vi "ElevatorStateControl.vi"(9 "Elevator State":string) -> (1 "Elevator State Out":string, 2 "Target Elevator Position":dbl, 4 "Target Vacuum Pump Power":dbl)   [LabVIEW 2018]
uses:
  Inputs_DriverStation.vi
  SensorReadings.vi
  RobotStates.vi
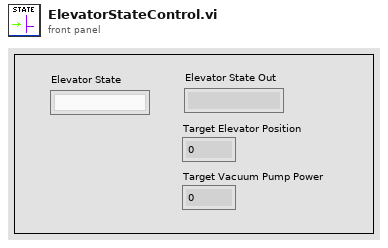
[diagram p1: front panel]
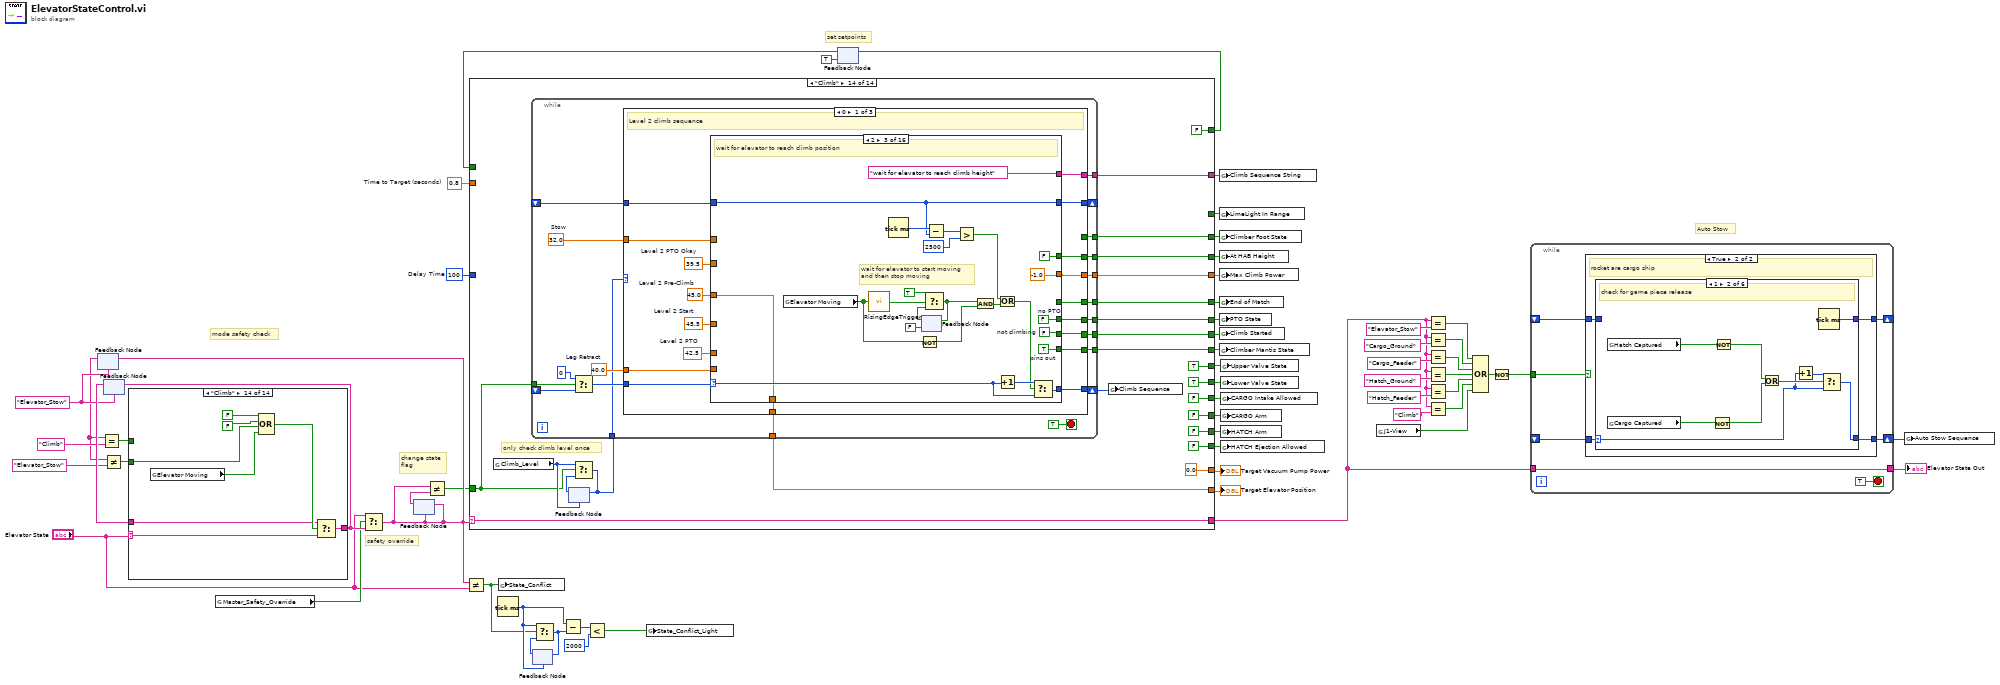
[diagram p0: block diagram]
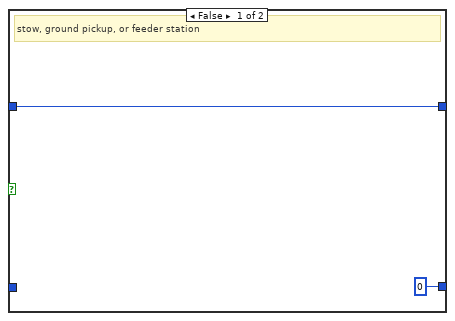
[diagram p2: hidden frame]
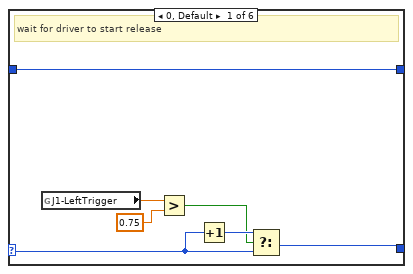
[diagram p3: hidden frame]
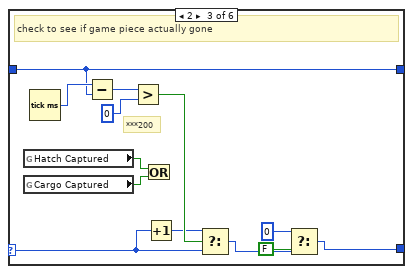
[diagram p4: hidden frame]
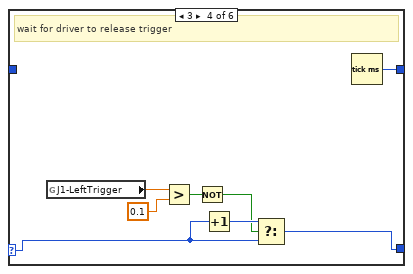
[diagram p5: hidden frame]
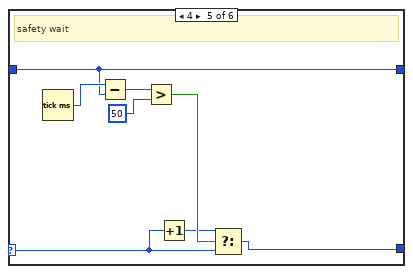
[diagram p6: hidden frame]
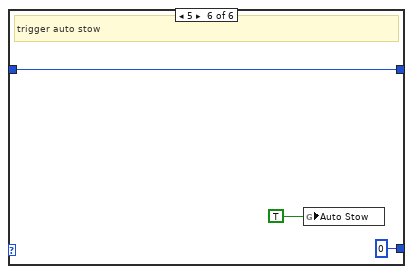
[diagram p7: hidden frame]
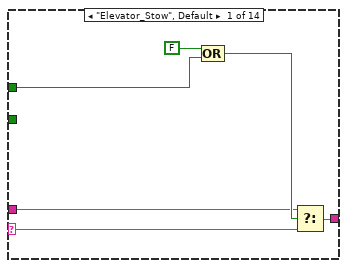
[diagram p8: hidden frame]
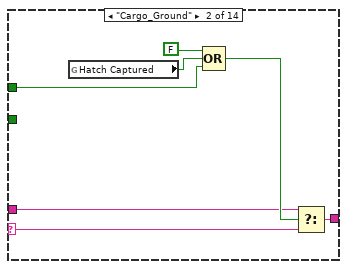
[diagram p9: hidden frame]
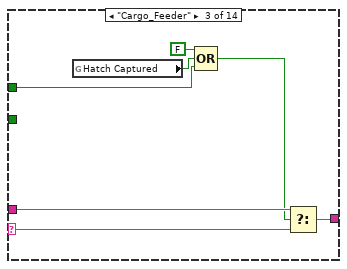
[diagram p10: hidden frame]
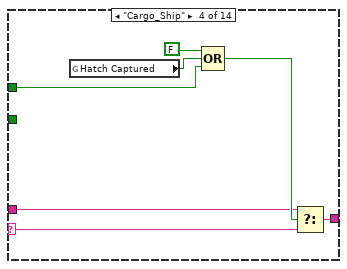
[diagram p11: hidden frame]
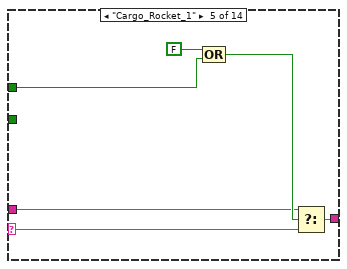
[diagram p12: hidden frame]
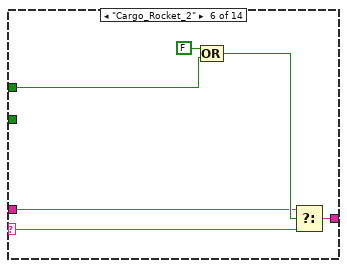
[diagram p13: hidden frame]
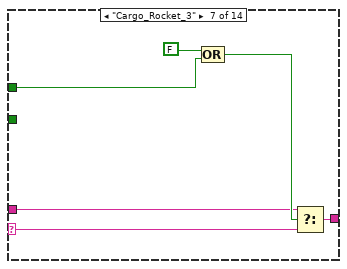
[diagram p14: hidden frame]
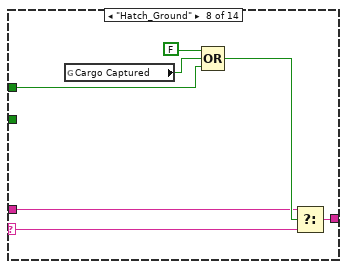
[diagram p15: hidden frame]
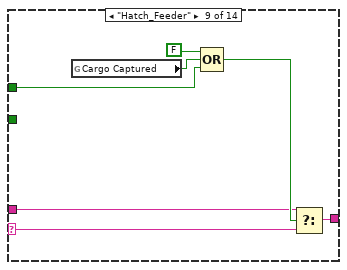
[diagram p16: hidden frame]
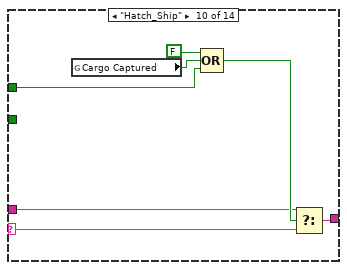
[diagram p17: hidden frame]
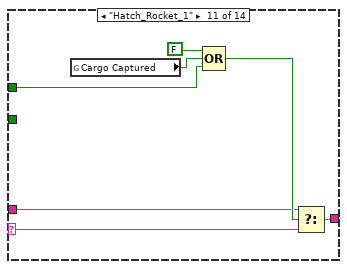
[diagram p18: hidden frame]
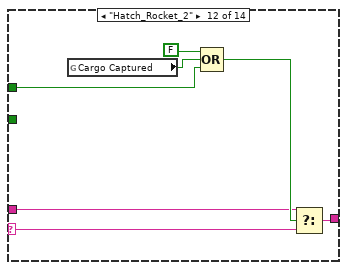
[diagram p19: hidden frame]
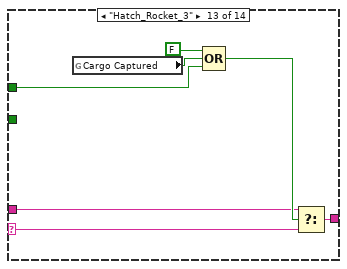
[diagram p20: hidden frame]
diagram:
  w3 = u32 100  # Delay Time
  w4 = 0.8  # Time to Target (seconds)
  w46 = "Elevator_Stow" ("Elevator State")
  # "change state\nflag"
  # "Auto Stow"
  # "safety override"
  # "mode safety check"
  # "set setpoints"
  n1 = feedback #1(w46) -> (w11:string)
  n2 = Equal?(x=w11, y="Climb") -> (x = y?=w47:bool)
  n3 = feedback #2(w46) -> (w49:string)
  n4 = Not Equal?(x=w11, y="Elevator_Stow") -> (x != y?=w10:bool)
  n5 = case shown="\"Climb\"" "Elevator State" {
    selector: "Elevator State" -> [w62 w69 w80 w83 w89 w95 w102 w108 w115 w122 w129 w136 w144 w152]
    tunnel: [w64 w71 w79 w85 w91 w97 w103 w110 w117 w124 w131 w138 w145 w153] -> w54
    tunnel: w49 -> [w63 w70 w78 w84 w90 w96 w101 w109 w116 w123 w130 w137 w143 w151]
    tunnel: w47 -> [w61 w67 w74 w81 w88 w94 w100 w106 w113 w120 w127 w134 w141 _]
    tunnel: w10 -> [_ _ _ _ _ _ _ _ _ _ _ _ _ w150]
    frame "Elevator_Stow", Default {
      n6 = Compound Arithmetic op=OR(FALSE, w61) -> (w65:bool)
      n7 = Select(t=w63, s=w65, f=w62) -> (s? t:f=w64:string)
    }
    frame "Cargo_Ground" {
      n8 = global read "SensorReadings.vi" "Hatch Captured"() -> (w68:bool)
      n9 = Compound Arithmetic op=OR(FALSE, w68, w67) -> (w72:bool)
      n10 = Select(t=w70, s=w72, f=w69) -> (s? t:f=w71:string)
    }
    frame "Cargo_Feeder" {
      n11 = global read "SensorReadings.vi" "Hatch Captured"() -> (w75:bool)
      n12 = Compound Arithmetic op=OR(FALSE, w75, w74) -> (w76:bool)
      n13 = Select(t=w78, s=w76, f=w80) -> (s? t:f=w79:string)
    }
    frame "Cargo_Ship" {
      n14 = global read "SensorReadings.vi" "Hatch Captured"() -> (w82:bool)
      n15 = Compound Arithmetic op=OR(FALSE, w82, w81) -> (w86:bool)
      n16 = Select(t=w84, s=w86, f=w83) -> (s? t:f=w85:string)
    }
    frame "Cargo_Rocket_1" {
      n17 = Compound Arithmetic op=OR(FALSE, w88) -> (w92:bool)
      n18 = Select(t=w90, s=w92, f=w89) -> (s? t:f=w91:string)
    }
    frame "Cargo_Rocket_2" {
      n19 = Compound Arithmetic op=OR(FALSE, w94) -> (w98:bool)
      n20 = Select(t=w96, s=w98, f=w95) -> (s? t:f=w97:string)
    }
    frame "Cargo_Rocket_3" {
      n21 = Compound Arithmetic op=OR(FALSE, w100) -> (w104:bool)
      n22 = Select(t=w101, s=w104, f=w102) -> (s? t:f=w103:string)
    }
    frame "Hatch_Ground" {
      n23 = global read "SensorReadings.vi" "Cargo Captured"() -> (w107:bool)
      n24 = Compound Arithmetic op=OR(FALSE, w107, w106) -> (w111:bool)
      n25 = Select(t=w109, s=w111, f=w108) -> (s? t:f=w110:string)
    }
    frame "Hatch_Feeder" {
      n26 = global read "SensorReadings.vi" "Cargo Captured"() -> (w114:bool)
      n27 = Compound Arithmetic op=OR(FALSE, w114, w113) -> (w118:bool)
      n28 = Select(t=w116, s=w118, f=w115) -> (s? t:f=w117:string)
    }
    frame "Hatch_Ship" {
      n29 = global read "SensorReadings.vi" "Cargo Captured"() -> (w121:bool)
      n30 = Compound Arithmetic op=OR(FALSE, w121, w120) -> (w125:bool)
      n31 = Select(t=w123, s=w125, f=w122) -> (s? t:f=w124:string)
    }
    frame "Hatch_Rocket_1" {
      n32 = global read "SensorReadings.vi" "Cargo Captured"() -> (w128:bool)
      n33 = Compound Arithmetic op=OR(FALSE, w128, w127) -> (w132:bool)
      n34 = Select(t=w130, s=w132, f=w129) -> (s? t:f=w131:string)
    }
    frame "Hatch_Rocket_2" {
      n35 = global read "SensorReadings.vi" "Cargo Captured"() -> (w135:bool)
      n36 = Compound Arithmetic op=OR(FALSE, w135, w134) -> (w139:bool)
      n37 = Select(t=w137, s=w139, f=w136) -> (s? t:f=w138:string)
    }
    frame "Hatch_Rocket_3" {
      n38 = global read "SensorReadings.vi" "Cargo Captured"() -> (w142:bool)
      n39 = Compound Arithmetic op=OR(FALSE, w142, w141) -> (w146:bool)
      n40 = Select(t=w143, s=w146, f=w144) -> (s? t:f=w145:string)
    }
    frame "Climb" {
      n41 = global read "RobotStates.vi" "Elevator Moving"() -> (w149:bool)
      n42 = Compound Arithmetic op=OR(FALSE, FALSE ("Cargo Captured"), w150, w149) -> (w154:bool)
      n43 = Select(t=w151, s=w154, f=w152) -> (s? t:f=w153:string)
    }
  }
  n44 = feedback-in #2(w54) -> ()
  n45 = global read "Inputs_DriverStation.vi" "Master_Safety_Override"() -> (w53:bool)
  n46 = Select(t="Elevator State", s=w53, f=w54) -> (s? t:f=w16:string)
  n47 = feedback-in #1(w16) -> ()
  n48 = feedback-in #3(w16) -> ()
  n49 = feedback #3(w16) -> (w17:string)
  n50 = Not Equal?(x=w16, y=w17) -> (x != y?=w15:bool)
  n51 = Not Equal?(x=w16, y="Elevator State") -> (x != y?=w22:bool)
  n52 = Tick Count (ms)() -> (millisecond timer value=w26:u32)
  n53 = global write "RobotStates.vi" "State_Conflict"(w22) -> ()
  n54 = feedback #4(w26) -> (w27:u32)
  n55 = Select(t=w26, s=w22, f=w27) -> (s? t:f=w25:u32)
  n56 = feedback-in #4(w25) -> ()
  n57 = Subtract(x=w26, y=w25) -> (x-y=w24:u32)
  n58 = Less?(x=w24, y=u32 2000) -> (x < y?=w21:bool)
  n59 = global write "RobotStates.vi" "State_Conflict_Light"(w21) -> ()
  n60 = feedback #5(TRUE) -> (w19:bool)
  n61 = case shown="\"Climb\"" w16 {
    selector: w16 -> [w179 w194 w234 w252 w293 w315 w337 w351 w413 w454 w495 w510 w525 w550]
    tunnel: [FALSE TRUE TRUE TRUE TRUE TRUE TRUE FALSE FALSE FALSE FALSE FALSE FALSE FALSE] -> w60
    tunnel: [w179 w194 w234 w252 w293 w315 w337 w351 w413 w454 w495 w510 w525 w550] -> w29
    tunnel: [w157 FALSE w197 w235 TRUE w296 w319 FALSE FALSE FALSE FALSE FALSE FALSE FALSE] -> w59
    tunnel: [w178 32.0 w204 w236 w279 w300 w317 32.0 w378 w440 w481 61.5 91.0 w536] -> w58
    tunnel: [FALSE FALSE FALSE FALSE FALSE FALSE FALSE TRUE w382 TRUE TRUE TRUE TRUE FALSE] -> w57
    tunnel: [w170 0.0 0.0 0.0 0.0 0.0 0.0 w347 w411 w452 w493 w506 w521 0.0 ("Vacuum_Pump")] -> w55
    tunnel: [FALSE FALSE FALSE FALSE FALSE FALSE FALSE TRUE TRUE TRUE TRUE TRUE TRUE FALSE] -> w56
    tunnel: [TRUE TRUE TRUE TRUE TRUE TRUE TRUE TRUE FALSE FALSE FALSE FALSE FALSE TRUE] -> w52
    tunnel: [TRUE TRUE TRUE TRUE TRUE TRUE TRUE FALSE TRUE TRUE TRUE TRUE TRUE TRUE] -> w51
    tunnel: [FALSE FALSE FALSE FALSE FALSE FALSE FALSE FALSE FALSE FALSE FALSE FALSE FALSE w539] -> w1
    tunnel: [w168 FALSE FALSE FALSE FALSE FALSE FALSE FALSE FALSE FALSE FALSE FALSE FALSE FALSE] -> w20
    tunnel: w19 -> [w164 _ _ _ _ _ _ _ _ _ _ _ _ _]
    tunnel: w15 -> [_ _ w212 _ _ _ _ _ w384 _ _ _ _ w538]
    tunnel: [w167 w184 w203 w244 w284 w307 w329 w342 w390 w447 w488 w501 w516 w535] -> w14
    tunnel: [w166 w183 w202 w243 w283 w306 w328 w341 w389 w446 w487 w500 w515 w534] -> w13
    tunnel: [FALSE FALSE FALSE FALSE FALSE FALSE FALSE FALSE FALSE FALSE FALSE FALSE FALSE w533] -> w9
    tunnel: [_ _ _ _ _ _ _ _ _ _ _ _ _ w531] -> w8
    tunnel: [-1.0 ("y") -1.0 ("y") -1.0 ("y") -1.0 ("y") -1.0 ("y") -1.0 ("y") -1.0 ("y") -1.0 ("y") -1.0 ("y") -1.0 ("y") -1.0 ("y") -1.0 ("y") -1.0 ("y") w530] -> w7
    tunnel: [_ _ _ _ _ _ _ _ _ _ _ _ _ w529] -> w6
    tunnel: [_ _ _ _ w271 _ _ _ w371 w433 w474 _ _ _] -> w5
    tunnel: w4 -> [_ _ _ _ w269 _ _ _ w369 w432 w472 _ _ _]
    tunnel: w3 -> [_ _ _ _ w270 _ _ _ w370 w431 w473 _ _ _]
    tunnel: [_ _ _ _ _ _ _ _ _ _ _ _ _ w528] -> w2
    frame "Elevator_Stow", Default {
      w166 = FALSE  # no PTO
      w167 = FALSE  # not climbing
      w178 = 30.0  # below 34.5 to ensure reset
      n62 = global read "Inputs_DriverStation.vi" "Reinit_Stow_Vacuum"() -> (w161:bool)
      n63 = global read "Inputs_DriverStation.vi" "Vacuum_Pump"() -> (w172:dbl)
      n64 = global read "RobotStates.vi" "Autopilot"() -> (w160:bool)
      n65 = Select(t=TRUE, s=w161, f=w164) -> (s? t:f=w163:bool)
      n66 = Select(t=w172, s=w163, f=0.0) -> (s? t:f=w170:dbl)
      n67 = Select(t=TRUE, s=w163, f=w163) -> (s? t:f=w168:bool)
      n68 = Select(t=TRUE, s=w160, f=FALSE) -> (s? t:f=w157:bool)
    }
    frame "Cargo_Ground" {
      w183 = FALSE  # no PTO
      w184 = FALSE  # not climbing
    }
    frame "Cargo_Feeder" {
      w199 = TRUE  # hold CARGO arm up
      w202 = FALSE  # no PTO
      w203 = FALSE  # not climbing
      w205 = 32.0  # gotten CARGO
      w209 = FALSE  # gotten CARGO
      w221 = -2.0  # (ft/s)
      w208 = 52.0  # getting CARGO
      w210 = TRUE  # getting CARGO
      # "autopilot"
      # "auto protect CARGO"
      n69 = global read "SensorReadings.vi" "EncoderVel_RightDrive"() -> (w225:dbl)
      n70 = global read "SensorReadings.vi" "EncoderVel_LeftDrive"() -> (w226:dbl)
      n71 = global read "SensorReadings.vi" "Cargo Captured"() -> (w219:bool)
      n72 = Add(x=w226, y=w225) -> (x+y=w224:dbl)
      n73 = Divide(x=w224, y=2.0) -> (x/y=w222:dbl)
      n74 = Less?(x=w222, y=w221) -> (x < y?=w220:bool)
      n75 = And(x=w220, y=w219) -> (x .and. y?=w218:bool)
      n76 = feedback #6(FALSE) -> (w216:bool)
      n77 = Select(t=TRUE, s=w218, f=w216) -> (s? t:f=w214:bool)
      n78 = Select(t=FALSE, s=w212, f=w214) -> (s? t:f=w207:bool)
      n79 = feedback-in #6(w207) -> ()
      n80 = Not(x=w207) -> (.not. x?=w206:bool)
      n81 = global read "RobotStates.vi" "Autopilot"() -> (w200:bool)
      n82 = Select(t=w210, s=w206, f=w209) -> (s? t:f=w198:bool)
      n83 = Select(t=w199, s=w200, f=w198) -> (s? t:f=w197:bool)
      n84 = Select(t=w208, s=w206, f=w205) -> (s? t:f=w204:dbl)
    }
    frame "Cargo_Ship" {
      w243 = FALSE  # no PTO
      w244 = FALSE  # not climbing
      w236 = 48.0
      # "46"
      n85 = global read "SensorReadings.vi" "EncoderPos_Elevator"() -> (w240:dbl)
      n86 = Subtract(x=w240, y=w236) -> (x-y=w239:dbl)
      n87 = Absolute Value(x=w239) -> (abs(x)=w237:dbl)
      n88 = Less?(x=w237, y=5.0) -> (x < y?=w235:bool)
    }
    frame "Cargo_Rocket_1" {
      w260 = 3.0  # feet per second
      w283 = FALSE  # no PTO
      w284 = FALSE  # not climbing
      n89 = global read "SensorReadings.vi" "LimeLight Distance (in)"() -> (w258:dbl)
      n90 = global read "SensorReadings.vi" "EncoderVel_RightDrive"() -> (w267:dbl)
      n91 = global read "SensorReadings.vi" "EncoderVel_LeftDrive"() -> (w268:dbl)
      n92 = Add(x=w268, y=w267) -> (x+y=w266:dbl)
      n93 = Divide(x=w258, y=12.0) -> (x/y=w256:dbl)
      n94 = Divide(x=w266, y=2.0) -> (x/y=w261:dbl)
      n95 = In Range and Coerce(upper limit=10.0, x=w261, lower limit=w260) -> (coerced(x)=w259:dbl)  [unwired: 1 out]
      n96 = Divide(x=w256, y=w259) -> (x/y=w263:dbl)
      n97 = Greater Than 0?(x=w263) -> (x > 0?=w264:bool)
      n98 = Select(t=w263, s=w264, f=inf) -> (s? t:f=w255:dbl)
      n99 = global read "SensorReadings.vi" "LimeLight Valid"() -> (w274:bool)
      n100 = Select(t=w255, s=w274, f=inf) -> (s? t:f=w273:dbl)
      n101 = call "TimeBelowThreshold.vi"("Current Value"=w273, "Threshold"=w269) -> ("Time Below"=w275:u32)  [unwired: 3 in]
      n102 = global read "RobotStates.vi" "Autopilot"() -> (w281:bool)
      n103 = Greater?(x=w275, y=w270) -> (0:w276:bool)
      n104 = call "RisingEdgeTrigger.vi"("Raw Signal"=w276) -> ("Trigger"=w271:bool)
      n105 = Select(t=45.0, s=w281, f=32.0) -> (s? t:f=w279:dbl)
    }
    frame "Cargo_Rocket_2" {
      w306 = FALSE  # no PTO
      w307 = FALSE  # not climbing
      w300 = 62.5
      n106 = global read "SensorReadings.vi" "EncoderPos_Elevator"() -> (w301:dbl)
      n107 = Subtract(x=w301, y=w300) -> (x-y=w299:dbl)
      n108 = Absolute Value(x=w299) -> (abs(x)=w295:dbl)
      n109 = Less?(x=w295, y=10.0) -> (x < y?=w297:bool)
      n110 = Select(t=TRUE, s=w297, f=FALSE) -> (s? t:f=w296:bool)
    }
    frame "Cargo_Rocket_3" {
      w328 = FALSE  # no PTO
      w329 = FALSE  # not climbing
      w317 = 91.0
      n111 = global read "SensorReadings.vi" "EncoderPos_Elevator"() -> (w323:dbl)
      n112 = Subtract(x=w323, y=w317) -> (x-y=w322:dbl)
      n113 = Absolute Value(x=w322) -> (abs(x)=w320:dbl)
      n114 = Less?(x=w320, y=10.0) -> (x < y?=w321:bool)
      n115 = Select(t=TRUE, s=w321, f=FALSE) -> (s? t:f=w319:bool)
    }
    frame "Hatch_Ground" {
      w341 = FALSE  # no PTO
      w342 = FALSE  # not climbing
      n116 = global read "Inputs_DriverStation.vi" "Vacuum_Pump"() -> (w347:dbl)
    }
    frame "Hatch_Feeder" {
      w359 = 3.0  # feet per second
      w389 = FALSE  # no PTO
      w390 = FALSE  # not climbing
      w400 = -2.0  # (ft/s)
      w392 = FALSE  # gotten HATCH
      w406 = TRUE  # to get HATCH
      # "auto protect HATCH"
      n117 = global read "SensorReadings.vi" "EncoderVel_RightDrive"() -> (w404:dbl)
      n118 = global read "SensorReadings.vi" "EncoderVel_LeftDrive"() -> (w405:dbl)
      n119 = global read "SensorReadings.vi" "LimeLight Distance (in)"() -> (w357:dbl)
      n120 = global read "SensorReadings.vi" "EncoderVel_RightDrive"() -> (w367:dbl)
      n121 = global read "SensorReadings.vi" "EncoderVel_LeftDrive"() -> (w368:dbl)
      n122 = global read "SensorReadings.vi" "Hatch Captured"() -> (w386:bool)
      n123 = Add(x=w405, y=w404) -> (x+y=w403:dbl)
      n124 = Divide(x=w403, y=2.0) -> (x/y=w401:dbl)
      n125 = Less?(x=w401, y=w400) -> (x < y?=w399:bool)
      n126 = Add(x=w368, y=w367) -> (x+y=w366:dbl)
      n127 = And(x=w399, y=w386) -> (x .and. y?=w398:bool)
      n128 = Not(x=w386) -> (.not. x?=w385:bool)
      n129 = Divide(x=w357, y=12.0) -> (x/y=w355:dbl)
      n130 = Divide(x=w366, y=2.0) -> (x/y=w360:dbl)
      n131 = Or(x=w385, y=w384) -> (x .or. y?=w383:bool)
      n132 = feedback #7(FALSE) -> (w396:bool)
      n133 = Select(t=TRUE, s=w398, f=w396) -> (s? t:f=w394:bool)
      n134 = In Range and Coerce(upper limit=10.0 ("feet per second"), x=w360, lower limit=w359) -> (coerced(x)=w358:dbl)  [unwired: 1 out]
      n135 = Select(t=FALSE, s=w383, f=w394) -> (s? t:f=w391:bool)
      n136 = feedback-in #7(w391) -> ()
      n137 = Divide(x=w355, y=w358) -> (x/y=w363:dbl)
      n138 = Not(x=w391) -> (.not. x?=w387:bool)
      n139 = Greater Than 0?(x=w363) -> (x > 0?=w364:bool)
      n140 = Select(t=w363, s=w364, f=inf) -> (s? t:f=w361:dbl)
      n141 = global read "SensorReadings.vi" "LimeLight Valid"() -> (w375:bool)
      n142 = Select(t=w406, s=w387, f=w392) -> (s? t:f=w382:bool)
      n143 = Select(t=w361, s=w375, f=inf) -> (s? t:f=w376:dbl)
      n144 = global read "RobotStates.vi" "Autopilot"() -> (w381:bool)
      n145 = call "TimeBelowThreshold.vi"("Current Value"=w376, "Threshold"=w369) -> ("Time Below"=w373:u32)  [unwired: 3 in]
      n146 = global read "Inputs_DriverStation.vi" "Vacuum_Pump"() -> (w411:dbl)
      n147 = Greater?(x=w373, y=w370) -> (0:w372:bool)
      n148 = Select(t=55.0, s=w381, f=32.0) -> (s? t:f=w378:dbl)
      n149 = call "RisingEdgeTrigger.vi"("Raw Signal"=w372) -> ("Trigger"=w371:bool)
    }
    frame "Hatch_Ship" {
      w422 = 3.0  # feet per second
      w446 = FALSE  # no PTO
      w447 = FALSE  # not climbing
      n150 = global read "SensorReadings.vi" "LimeLight Distance (in)"() -> (w420:dbl)
      n151 = global read "SensorReadings.vi" "EncoderVel_RightDrive"() -> (w429:dbl)
      n152 = global read "SensorReadings.vi" "EncoderVel_LeftDrive"() -> (w430:dbl)
      n153 = Add(x=w430, y=w429) -> (x+y=w428:dbl)
      n154 = Divide(x=w420, y=12.0) -> (x/y=w418:dbl)
      n155 = Divide(x=w428, y=2.0) -> (x/y=w423:dbl)
      n156 = In Range and Coerce(upper limit=10.0, x=w423, lower limit=w422) -> (coerced(x)=w421:dbl)  [unwired: 1 out]
      n157 = Divide(x=w418, y=w421) -> (x/y=w425:dbl)
      n158 = Greater Than 0?(x=w425) -> (x > 0?=w426:bool)
      n159 = Select(t=w425, s=w426, f=inf) -> (s? t:f=w417:dbl)
      n160 = global read "SensorReadings.vi" "LimeLight Valid"() -> (w437:bool)
      n161 = Select(t=w417, s=w437, f=inf) -> (s? t:f=w438:dbl)
      n162 = call "TimeBelowThreshold.vi"("Current Value"=w438, "Threshold"=w432) -> ("Time Below"=w435:u32)  [unwired: 3 in]
      n163 = global read "RobotStates.vi" "Autopilot"() -> (w443:bool)
      n164 = global read "Inputs_DriverStation.vi" "Vacuum_Pump"() -> (w452:dbl)
      n165 = Greater?(x=w435, y=w431) -> (0:w434:bool)
      n166 = call "RisingEdgeTrigger.vi"("Raw Signal"=w434) -> ("Trigger"=w433:bool)
      n167 = Select(t=55.0, s=w443, f=32.0) -> (s? t:f=w440:dbl)
    }
    frame "Hatch_Rocket_1" {
      w463 = 3.0  # feet per second
      w487 = FALSE  # no PTO
      w488 = FALSE  # not climbing
      # "autopilot"
      n168 = global read "SensorReadings.vi" "LimeLight Distance (in)"() -> (w461:dbl)
      n169 = global read "SensorReadings.vi" "EncoderVel_RightDrive"() -> (w470:dbl)
      n170 = global read "SensorReadings.vi" "EncoderVel_LeftDrive"() -> (w471:dbl)
      n171 = Add(x=w471, y=w470) -> (x+y=w469:dbl)
      n172 = Divide(x=w461, y=12.0) -> (x/y=w459:dbl)
      n173 = Divide(x=w469, y=2.0) -> (x/y=w464:dbl)
      n174 = In Range and Coerce(upper limit=10.0, x=w464, lower limit=w463) -> (coerced(x)=w462:dbl)  [unwired: 1 out]
      n175 = Divide(x=w459, y=w462) -> (x/y=w466:dbl)
      n176 = Greater Than 0?(x=w466) -> (x > 0?=w467:bool)
      n177 = Select(t=w466, s=w467, f=inf) -> (s? t:f=w458:dbl)
      n178 = global read "SensorReadings.vi" "LimeLight Valid"() -> (w477:bool)
      n179 = Select(t=w458, s=w477, f=inf) -> (s? t:f=w476:dbl)
      n180 = call "TimeBelowThreshold.vi"("Current Value"=w476, "Threshold"=w472) -> ("Time Below"=w478:u32)  [unwired: 3 in]
      n181 = Greater?(x=w478, y=w473) -> (0:w479:bool)
      n182 = global read "RobotStates.vi" "Autopilot"() -> (w484:bool)
      n183 = global read "Inputs_DriverStation.vi" "Vacuum_Pump"() -> (w493:dbl)
      n184 = call "RisingEdgeTrigger.vi"("Raw Signal"=w479) -> ("Trigger"=w474:bool)
      n185 = Select(t=55.0, s=w484, f=32.0) -> (s? t:f=w481:dbl)
    }
    frame "Hatch_Rocket_2" {
      w500 = FALSE  # no PTO
      w501 = FALSE  # not climbing
      n186 = global read "Inputs_DriverStation.vi" "Vacuum_Pump"() -> (w506:dbl)
    }
    frame "Hatch_Rocket_3" {
      w515 = FALSE  # no PTO
      w516 = FALSE  # not climbing
      n187 = global read "Inputs_DriverStation.vi" "Vacuum_Pump"() -> (w521:dbl)
    }
    frame "Climb" {
      # "only check climb level once"
      n188 = global read "Inputs_DriverStation.vi" "Climb_Level"() -> (w540:u8)
      n189 = feedback #8(w540) -> (w541:u8)
      n190 = Select(t=w540, s=w538, f=w541) -> (s? t:f=w537:u8)
      n191 = while {
        shift-right: [w569] -> w532
        shift-left: _ -> [w565]
        shift-right: [w568] -> _
        shift-left: _ -> [w567]
        tunnel: [w566] -> w539
        tunnel: w538 -> [w563]
        tunnel: w537 -> [w556]
        tunnel: [w558] -> w536
        tunnel: [w561] -> w535
        tunnel: [w560] -> w534
        tunnel: [w559] -> w533
        tunnel: [w555] -> w531
        tunnel: [w554] -> w530
        tunnel: [w553] -> w529
        tunnel: [w551] -> w528
        stop <- TRUE stop-if-true
        w552 = 32.0  # Stow
        w557 = 40.0  # Leg Retract
        n192 = Select(t=0, s=w563, f=w565) -> (s? t:f=w564:i32)
        n193 = case shown="0" w556 {
          tunnel: [w582 w841 w1064] -> w569
          tunnel: [w586 w848 w1071] -> w568
          tunnel: w567 -> [w588 w849 w1072]
          tunnel: [w581 w842 w1065] -> w566
          tunnel: w564 -> [w584 w847 w1070]
          tunnel: [w579 w843 w1066] -> w561
          tunnel: [w580 w844 w1067] -> w560
          tunnel: [w583 w845 w1068] -> w559
          tunnel: [w578 w840 w1063] -> w558
          tunnel: w557 -> [w585 w846 w1069]
          tunnel: [w587 w839 w1062] -> w555
          tunnel: [w577 w837 w1060] -> w554
          tunnel: [w576 w835 w1058] -> w553
          tunnel: w552 -> [w571 w834 w1057]
          tunnel: [_ _ w1056] -> w551
          frame 0 {
            w575 = 45.0  # Level 2 Pre-Climb
            w572 = 39.5  # Level 2 PTO Okay
            w574 = 45.5  # Level 2 Start
            w573 = 42.5  # Level 2 PTO
            # "Level 2 climb sequence"
            n194 = case shown="2" w584 {
              selector: w584 -> [w598 w614 w634 w651 w662 w683 w694 w713 w732 w743 w761 w770 w785 w797 w814 w828]
              tunnel: [w600 w616 w630 w650 w661 w682 w696 w715 w731 w742 w760 w769 w784 w796 w813 w828] -> w582
              tunnel: [w597 w601 w620 w648 w664 w675 w695 w714 w727 w735 w748 w773 w787 w799 w821 w831] -> w586
              tunnel: w588 -> [_ w604 w620 _ w664 w675 w695 w714 w727 _ w748 w773 w787 w799 w821 w831]
              tunnel: [w596 w613 w640 w649 w660 w685 w699 w718 w734 w745 w763 w774 w788 w800 w822 w832] -> w581
              tunnel: [w589 w602 w624 w641 w653 w668 _ w703 _ _ _ _ w780 w795 w816 w825] -> w578
              tunnel: [w594 w612 w629 w646 w659 w678 w700 w719 w730 w741 w759 w775 w789 w801 w823 w833] -> w579
              tunnel: [w593 w611 w628 w645 w658 w677 w701 w720 w729 w740 w758 w768 w783 w793 w819 w829] -> w580
              tunnel: [FALSE FALSE FALSE FALSE FALSE FALSE FALSE FALSE FALSE FALSE FALSE w772 TRUE TRUE TRUE FALSE] -> w583
              tunnel: w585 -> [_ _ _ _ _ _ _ _ _ _ _ _ w780 w795 w816 w825]
              tunnel: ["release mantis" "wait for mantis to deploy" "wait for elevator to reach climb height" "lock mantis" "confirm mantis lock" "wait for the driver to start climbing #1" "wait for driver to raise elevator" "wait for elevator to reach start height" "wait for elevator to pass PTO height" "engage the PTO" "ensure PTO is engaged" "wait for the robot to be on HAB" "stop climbing" "wait to disengage PTO" "retract the legs after confirm " "elevator powered down"] -> w587
              tunnel: [-1.0 ("y") -1.0 ("y") -1.0 ("y") -1.0 ("y") -1.0 ("y") -1.0 ("y") -1.0 ("y") -1.0 ("y") -0.05 ("y") -0.05 ("y") -0.05 ("y") -1.0 ("y") -1.0 ("y") -1.0 ("y") -1.0 ("y") -1.0 ("y")] -> w577
              tunnel: [_ _ _ _ _ _ _ _ _ _ _ _ _ _ _ w824] -> w576
              tunnel: w575 -> [_ _ w624 w641 w653 w668 _ _ _ _ _ _ _ _ _ _]
              tunnel: w574 -> [_ _ _ _ _ _ _ w703 _ _ _ _ _ _ _ _]
              tunnel: w573 -> [_ _ _ _ _ _ _ _ w722 _ _ _ _ _ _ _]
              tunnel: w572 -> [_ _ _ _ _ _ _ _ _ _ w746 _ _ _ _ _]
              tunnel: w571 -> [w589 w602 _ _ _ _ _ _ _ _ _ _ _ _ _ _]
              frame 0, Default {
                w593 = FALSE  # no PTO
                w594 = FALSE  # not climbing
                w596 = TRUE  # pins out
                # "release mantis pins and command to climb height"
                n195 = Increment(x=w598) -> (x+1=w599:i32)
                n196 = Select(t=w599, s=TRUE, f=w598) -> (s? t:f=w600:i32)
                n197 = Tick Count (ms)() -> (millisecond timer value=w597:u32)
              }
              frame 1 {
                w611 = FALSE  # no PTO
                w612 = FALSE  # not climbing
                w613 = TRUE  # pins out
                # "wait for mantis to deploy"
                n198 = Tick Count (ms)() -> (millisecond timer value=w607:u32)
                n199 = Subtract(x=w607, y=w604) -> (x-y=w606:u32)
                n200 = Greater?(x=w606, y=u32 0) -> (0:w603:bool)
                n201 = Increment(x=w614) -> (x+1=w615:i32)
                n202 = Select(t=w615, s=w603, f=w614) -> (s? t:f=w616:i32)
                n203 = Tick Count (ms)() -> (millisecond timer value=w601:u32)
              }
              frame 2 {
                w628 = FALSE  # no PTO
                w629 = FALSE  # not climbing
                w640 = TRUE  # pins out
                # "wait for elevator to start moving\nand then stop moving"
                # "wait for elevator to reach climb position"
                n204 = global read "RobotStates.vi" "Elevator Moving"() -> (w632:bool)
                n205 = call "RisingEdgeTrigger.vi"("Raw Signal"=w632) -> ("Trigger"=w639:bool)
                n206 = Tick Count (ms)() -> (millisecond timer value=w623:u32)
                n207 = Not(x=w632) -> (.not. x?=w631:bool)
                n208 = feedback #9(FALSE) -> (w637:bool)
                n209 = Select(t=TRUE, s=w639, f=w637) -> (s? t:f=w633:bool)
                n210 = feedback-in #9(w633) -> ()
                n211 = Subtract(x=w623, y=w620) -> (x-y=w622:u32)
                n212 = Greater?(x=w622, y=u32 2500) -> (0:w617:bool)
                n213 = And(x=w633, y=w631) -> (x .and. y?=w619:bool)
                n214 = Or(x=w617, y=w619) -> (x .or. y?=w618:bool)
                n215 = Increment(x=w634) -> (x+1=w635:i32)
                n216 = Select(t=w635, s=w618, f=w634) -> (s? t:f=w630:i32)
              }
              frame 3 {
                w645 = FALSE  # no PTO
                w646 = FALSE  # not climbing
                w649 = FALSE  # pins in
                # "lock mantis pins"
                n217 = Increment(x=w651) -> (x+1=w652:i32)
                n218 = Tick Count (ms)() -> (millisecond timer value=w648:u32)
                n219 = Select(t=w652, s=TRUE, f=w651) -> (s? t:f=w650:i32)
              }
              frame 4 {
                w658 = FALSE  # no PTO
                w659 = FALSE  # not climbing
                w660 = FALSE  # pins in
                # "wait for mantis legs to lock"
                n220 = Tick Count (ms)() -> (millisecond timer value=w667:u32)
                n221 = Subtract(x=w667, y=w664) -> (x-y=w666:u32)
                n222 = Greater?(x=w666, y=u32 500) -> (0:w656:bool)
                n223 = Increment(x=w662) -> (x+1=w663:i32)
                n224 = Select(t=w663, s=w656, f=w662) -> (s? t:f=w661:i32)
              }
              frame 5 {
                w677 = FALSE  # no PTO
                w678 = FALSE  # not climbing
                w685 = FALSE  # pins in
                # "wait for the driver to start climbing"
                n225 = global read "Inputs_DriverStation.vi" "J1-RightTrigger"() -> (w674:dbl)
                n226 = Greater?(x=w674, y=0.2) -> (0:w672:bool)
                n227 = feedback #10(FALSE) -> (w679:bool)
                n228 = Select(t=TRUE, s=w672, f=w679) -> (s? t:f=w671:bool)
                n229 = feedback-in #10(w671) -> ()
                n230 = Increment(x=w683) -> (x+1=w684:i32)
                n231 = Select(t=w684, s=w671, f=w683) -> (s? t:f=w682:i32)
              }
              frame 6 {
                w701 = FALSE  # no PTO
                w700 = TRUE  # climbing
                w699 = FALSE  # pins in
                # "Lower elevator contacts HAB first time"
                n232 = global read "Inputs_DriverStation.vi" "J1-LeftTrigger"() -> (w690:dbl)
                n233 = Greater?(x=w690, y=0.75) -> (0:w688:bool)
                n234 = feedback #11(FALSE) -> (w691:bool)
                n235 = Select(t=TRUE, s=w688, f=w691) -> (s? t:f=w687:bool)
                n236 = feedback-in #11(w687) -> ()
                n237 = Increment(x=w694) -> (x+1=w697:i32)
                n238 = Select(t=w697, s=w687, f=w694) -> (s? t:f=w696:i32)
              }
              frame 7 {
                w720 = FALSE  # no PTO
                w719 = FALSE  # not climbing
                w718 = FALSE  # pins in
                # "Wait for elevator to reach start height"
                n239 = global read "RobotStates.vi" "Elevator Moving"() -> (w706:bool)
                n240 = call "RisingEdgeTrigger.vi"("Raw Signal"=w706) -> ("Trigger"=w711:bool)
                n241 = Not(x=w706) -> (.not. x?=w705:bool)
                n242 = feedback #12(FALSE) -> (w709:bool)
                n243 = Select(t=TRUE, s=w711, f=w709) -> (s? t:f=w707:bool)
                n244 = feedback-in #12(w707) -> ()
                n245 = And(x=w707, y=w705) -> (x .and. y?=w704:bool)
                n246 = Increment(x=w713) -> (x+1=w716:i32)
                n247 = Select(t=w716, s=w704, f=w713) -> (s? t:f=w715:i32)
              }
              frame 8 {
                w729 = FALSE  # no PTO
                w730 = TRUE  # climbing
                w734 = FALSE  # pins in
                # "wait for elevator to pass PTO height"
                n248 = global read "SensorReadings.vi" "EncoderPos_Elevator"() -> (w723:dbl)
                n249 = Less Or Equal?(x=w723, y=w722) -> (x <= y?=w724:bool)
                n250 = Increment(x=w732) -> (x+1=w733:i32)
                n251 = Select(t=w733, s=w724, f=w732) -> (s? t:f=w731:i32)
              }
              frame 9 {
                w740 = TRUE  # PTO
                w741 = TRUE  # climbing
                w745 = FALSE  # pins in
                # "engage the PTO"
                n252 = Increment(x=w743) -> (x+1=w744:i32)
                n253 = Tick Count (ms)() -> (millisecond timer value=w735:u32)
                n254 = Select(t=w744, s=TRUE, f=w743) -> (s? t:f=w742:i32)
              }
              frame 10 {
                w758 = TRUE  # PTO
                w759 = TRUE  # climbing
                w763 = FALSE  # pins in
                # "timeout"
                # "ensure PTO is engaged"
                n255 = global read "SensorReadings.vi" "EncoderPos_Elevator"() -> (w754:dbl)
                n256 = Tick Count (ms)() -> (millisecond timer value=w751:u32)
                n257 = Less Or Equal?(x=w754, y=w746) -> (x <= y?=w753:bool)
                n258 = Subtract(x=w751, y=w748) -> (x-y=w750:u32)
                n259 = Greater?(x=w750, y=u32 1000) -> (0:w747:bool)
                n260 = Or(x=w747, y=w753) -> (x .or. y?=w752:bool)
                n261 = Increment(x=w761) -> (x+1=w762:i32)
                n262 = Select(t=w762, s=w752, f=w761) -> (s? t:f=w760:i32)
              }
              frame 11 {
                w768 = TRUE  # PTO
                w775 = TRUE  # climbing
                w774 = FALSE  # pins in
                # "wait for robot to be secure on HAB"
                n263 = global read "Inputs_DriverStation.vi" "Master_Safety_Override"() -> (w776:bool)
                n264 = global read "SensorReadings.vi" "Robot On Ground"() -> (w764:bool)
                n265 = global read "Inputs_DriverStation.vi" "J1-Menu"() -> (w777:bool)
                n266 = Or(x=w764, y=w776) -> (x .or. y?=w772:bool)
                n267 = And(x=w777, y=w772) -> (x .and. y?=w767:bool)
                n268 = Increment(x=w770) -> (x+1=w771:i32)
                n269 = Select(t=w771, s=w767, f=w770) -> (s? t:f=w769:i32)
              }
              frame 12 {
                w783 = TRUE  # PTO
                w789 = FALSE  # not climbing
                w788 = FALSE  # pins in
                # "stop \"climbing\""
                n270 = Increment(x=w785) -> (x+1=w786:i32)
                n271 = Select(t=w786, s=TRUE, f=w785) -> (s? t:f=w784:i32)
              }
              frame 13 {
                w793 = TRUE  # PTO
                w801 = FALSE  # not climbing
                w800 = FALSE  # pins in
                # "wait to disengage PTO"
                n272 = Increment(x=w797) -> (x+1=w798:i32)
                n273 = Select(t=w798, s=TRUE, f=w797) -> (s? t:f=w796:i32)
              }
              frame 14 {
                w819 = FALSE  # no PTO
                w823 = FALSE  # not climbing
                w822 = FALSE  # pins in
                # "retract legs"
                n274 = global read "Inputs_DriverStation.vi" "J1-Menu"() -> (w803:bool)
                n275 = Not(x=w803) -> (.not. x?=w804:bool)
                n276 = feedback #13(FALSE ("PTO")) -> (w807:bool)
                n277 = Select(t=TRUE ("no PTO"), s=w804, f=w807) -> (s? t:f=w802:bool)
                n278 = feedback-in #13(w802) -> ()
                n279 = And(x=w802, y=w803) -> (x .and. y?=w805:bool)
                n280 = feedback #14(FALSE ("PTO")) -> (w811:bool)
                n281 = Select(t=TRUE ("no PTO"), s=w805, f=w811) -> (s? t:f=w809:bool)
                n282 = feedback-in #14(w809) -> ()
                n283 = Increment(x=w814) -> (x+1=w815:i32)
                n284 = Select(t=w815, s=w809, f=w814) -> (s? t:f=w813:i32)
              }
              frame 15 {
                w824 = TRUE  # end of match
                w829 = FALSE  # no PTO
                w833 = FALSE  # not climbing
                w832 = FALSE  # pins in
                # "turn off the elevator"
              }
            }
          }
          frame 1, Default {
            w836 = 57.0  # Level 3 PTO Okay
            w838 = 62.0  # Level 3 Start
            w850 = 60.0  # Level 3 PTO
            # "Level 3 climb sequence"
            n285 = case shown="3" w847 {
              selector: w847 -> [w860 w875 w890 w907 w918 w939 w952 w964 w983 w992 w1007 w1019 w1036 w1050]
              tunnel: [w862 w877 w885 w906 w917 w938 w951 w963 w982 w991 w1006 w1018 w1035 w1050] -> w841
              tunnel: [w859 w865 w883 w904 w920 w931 w947 w955 w968 w995 w1009 w1021 w1043 w1053] -> w848
              tunnel: w849 -> [_ w865 w883 _ w920 w931 w947 _ w968 w995 w1009 w1021 w1043 w1053]
              tunnel: [w858 w874 w896 w905 w916 w941 w954 w966 w985 w996 w1010 w1022 w1044 w1054] -> w842
              tunnel: [w851 w863 w879 w898 w910 w925 _ w958 w978 _ w1002 w1017 w1038 w1047] -> w840
              tunnel: w850 -> [_ _ _ _ _ _ w944 w958 w978 _ _ _ _ _]
              tunnel: [w856 w873 w884 w902 w915 w934 w950 w962 w981 w997 w1011 w1023 w1045 w1055] -> w843
              tunnel: [w855 w872 w882 w901 w914 w933 w949 w961 w980 w990 w1005 w1015 w1041 w1051] -> w844
              tunnel: [FALSE FALSE FALSE FALSE FALSE FALSE FALSE FALSE FALSE w994 TRUE TRUE TRUE FALSE] -> w845
              tunnel: w846 -> [_ _ _ _ _ _ _ _ _ _ w1002 w1017 w1038 w1047]
              tunnel: ["release mantis" "wait for mantis to deploy" "wait for elevator to reach climb height" "lock mantis" "confirm mantis lock" "wait for the driver to start climbing" "wait for elevator to pass PTO height" "engage the PTO" "ensure PTO is engaged" "wait for the robot to be on HAB" "stop climbing" "wait to disengage PTO" "retract the legs after confirm " "elevator powered down"] -> w839
              tunnel: w838 -> [_ _ w879 w898 w910 w925 _ _ _ _ _ _ _ _]
              tunnel: [-1.0 ("y") -1.0 ("y") -1.0 ("y") -1.0 ("y") -1.0 ("y") -1.0 ("y") -0.05 ("y") -0.05 ("y") -0.05 ("y") -1.0 ("y") -1.0 ("y") -1.0 ("y") -1.0 ("y") -1.0 ("y")] -> w837
              tunnel: w836 -> [_ _ _ _ _ _ _ _ w974 _ _ _ _ _]
              tunnel: [_ _ _ _ _ _ _ _ _ _ _ _ _ w1046] -> w835
              tunnel: w834 -> [w851 w863 _ _ _ _ _ _ _ _ _ _ _ _]
              frame 0, Default {
                w855 = FALSE  # no PTO
                w856 = FALSE  # not climbing
                w858 = TRUE  # pins out
                # "release mantis pins and command to climb height"
                n286 = Increment(x=w860) -> (x+1=w861:i32)
                n287 = Select(t=w861, s=TRUE, f=w860) -> (s? t:f=w862:i32)
                n288 = Tick Count (ms)() -> (millisecond timer value=w859:u32)
              }
              frame 1 {
                w872 = FALSE  # no PTO
                w873 = FALSE  # not climbing
                w874 = TRUE  # pins out
                # "wait for mantis to deploy"
                n289 = Tick Count (ms)() -> (millisecond timer value=w868:u32)
                n290 = Subtract(x=w868, y=w865) -> (x-y=w867:u32)
                n291 = Greater?(x=w867, y=u32 250) -> (0:w864:bool)
                n292 = Increment(x=w875) -> (x+1=w876:i32)
                n293 = Select(t=w876, s=w864, f=w875) -> (s? t:f=w877:i32)
              }
              frame 2 {
                w882 = FALSE  # no PTO
                w884 = FALSE  # not climbing
                w896 = TRUE  # pins out
                # "wait for elevator to start moving\nand then stop moving"
                # "wait for elevator to reach climb position"
                n294 = global read "RobotStates.vi" "Elevator Moving"() -> (w888:bool)
                n295 = call "RisingEdgeTrigger.vi"("Raw Signal"=w888) -> ("Trigger"=w895:bool)
                n296 = Not(x=w888) -> (.not. x?=w887:bool)
                n297 = feedback #15(FALSE) -> (w893:bool)
                n298 = Select(t=TRUE, s=w895, f=w893) -> (s? t:f=w889:bool)
                n299 = feedback-in #15(w889) -> ()
                n300 = And(x=w889, y=w887) -> (x .and. y?=w886:bool)
                n301 = Increment(x=w890) -> (x+1=w891:i32)
                n302 = Select(t=w891, s=w886, f=w890) -> (s? t:f=w885:i32)
              }
              frame 3 {
                w901 = FALSE  # no PTO
                w902 = FALSE  # not climbing
                w905 = FALSE  # pins in
                # "lock mantis pins"
                n303 = Increment(x=w907) -> (x+1=w908:i32)
                n304 = Tick Count (ms)() -> (millisecond timer value=w904:u32)
                n305 = Select(t=w908, s=TRUE, f=w907) -> (s? t:f=w906:i32)
              }
              frame 4 {
                w914 = FALSE  # no PTO
                w915 = FALSE  # not climbing
                w916 = FALSE  # pins in
                # "wait for mantis legs to lock"
                n306 = Tick Count (ms)() -> (millisecond timer value=w923:u32)
                n307 = Subtract(x=w923, y=w920) -> (x-y=w922:u32)
                n308 = Greater?(x=w922, y=u32 500) -> (0:w912:bool)
                n309 = Increment(x=w918) -> (x+1=w919:i32)
                n310 = Select(t=w919, s=w912, f=w918) -> (s? t:f=w917:i32)
              }
              frame 5 {
                w933 = FALSE  # no PTO
                w934 = FALSE  # not climbing
                w941 = FALSE  # pins in
                # "wait for the driver to start climbing"
                n311 = global read "Inputs_DriverStation.vi" "J1-RightTrigger"() -> (w930:dbl)
                n312 = Greater?(x=w930, y=0.2) -> (0:w928:bool)
                n313 = feedback #16(FALSE) -> (w935:bool)
                n314 = Select(t=TRUE, s=w928, f=w935) -> (s? t:f=w927:bool)
                n315 = feedback-in #16(w927) -> ()
                n316 = Increment(x=w939) -> (x+1=w940:i32)
                n317 = Select(t=w940, s=w927, f=w939) -> (s? t:f=w938:i32)
              }
              frame 6 {
                w949 = FALSE  # no PTO
                w950 = TRUE  # climbing
                w954 = FALSE  # pins in
                # "wait for elevator to pass PTO height"
                n318 = global read "SensorReadings.vi" "EncoderPos_Elevator"() -> (w942:dbl)
                n319 = Less Or Equal?(x=w942, y=w944) -> (x <= y?=w943:bool)
                n320 = Increment(x=w952) -> (x+1=w953:i32)
                n321 = Select(t=w953, s=w943, f=w952) -> (s? t:f=w951:i32)
              }
              frame 7 {
                w961 = TRUE  # PTO
                w962 = TRUE  # climbing
                w966 = FALSE  # pins in
                # "engage the PTO"
                n322 = Increment(x=w964) -> (x+1=w965:i32)
                n323 = Tick Count (ms)() -> (millisecond timer value=w955:u32)
                n324 = Select(t=w965, s=TRUE, f=w964) -> (s? t:f=w963:i32)
              }
              frame 8 {
                w980 = TRUE  # PTO
                w981 = TRUE  # climbing
                w985 = FALSE  # pins in
                # "timeout"
                # "ensure PTO is engaged"
                n325 = global read "SensorReadings.vi" "EncoderPos_Elevator"() -> (w975:dbl)
                n326 = Tick Count (ms)() -> (millisecond timer value=w971:u32)
                n327 = Less Or Equal?(x=w975, y=w974) -> (x <= y?=w973:bool)
                n328 = Subtract(x=w971, y=w968) -> (x-y=w970:u32)
                n329 = Greater?(x=w970, y=u32 1000) -> (0:w967:bool)
                n330 = Or(x=w967, y=w973) -> (x .or. y?=w972:bool)
                n331 = Increment(x=w983) -> (x+1=w984:i32)
                n332 = Select(t=w984, s=w972, f=w983) -> (s? t:f=w982:i32)
              }
              frame 9 {
                w990 = TRUE  # PTO
                w997 = TRUE  # climbing
                w996 = FALSE  # pins in
                # "wait for robot to be secure on HAB"
                n333 = global read "Inputs_DriverStation.vi" "Master_Safety_Override"() -> (w998:bool)
                n334 = global read "SensorReadings.vi" "Robot On Ground"() -> (w986:bool)
                n335 = global read "Inputs_DriverStation.vi" "J1-Menu"() -> (w999:bool)
                n336 = Or(x=w986, y=w998) -> (x .or. y?=w994:bool)
                n337 = And(x=w999, y=w994) -> (x .and. y?=w989:bool)
                n338 = Increment(x=w992) -> (x+1=w993:i32)
                n339 = Select(t=w993, s=w989, f=w992) -> (s? t:f=w991:i32)
              }
              frame 10 {
                w1005 = TRUE  # PTO
                w1011 = FALSE  # not climbing
                w1010 = FALSE  # pins in
                # "stop \"climbing\""
                n340 = Increment(x=w1007) -> (x+1=w1008:i32)
                n341 = Select(t=w1008, s=TRUE, f=w1007) -> (s? t:f=w1006:i32)
              }
              frame 11 {
                w1015 = TRUE  # PTO
                w1023 = FALSE  # not climbing
                w1022 = FALSE  # pins in
                # "wait to disengage PTO"
                n342 = Increment(x=w1019) -> (x+1=w1020:i32)
                n343 = Select(t=w1020, s=TRUE, f=w1019) -> (s? t:f=w1018:i32)
              }
              frame 12 {
                w1041 = FALSE  # no PTO
                w1045 = FALSE  # not climbing
                w1044 = FALSE  # pins in
                # "retract legs"
                n344 = global read "Inputs_DriverStation.vi" "J1-Menu"() -> (w1025:bool)
                n345 = Not(x=w1025) -> (.not. x?=w1026:bool)
                n346 = feedback #17(FALSE ("PTO")) -> (w1029:bool)
                n347 = Select(t=TRUE ("no PTO"), s=w1026, f=w1029) -> (s? t:f=w1024:bool)
                n348 = feedback-in #17(w1024) -> ()
                n349 = And(x=w1024, y=w1025) -> (x .and. y?=w1027:bool)
                n350 = feedback #18(FALSE ("PTO")) -> (w1033:bool)
                n351 = Select(t=TRUE ("no PTO"), s=w1027, f=w1033) -> (s? t:f=w1031:bool)
                n352 = feedback-in #18(w1031) -> ()
                n353 = Increment(x=w1036) -> (x+1=w1037:i32)
                n354 = Select(t=w1037, s=w1031, f=w1036) -> (s? t:f=w1035:i32)
              }
              frame 13 {
                w1046 = TRUE  # end of match
                w1051 = FALSE  # no PTO
                w1055 = FALSE  # not climbing
                w1054 = FALSE  # pins in
                # "turn off the elevator"
              }
            }
          }
          frame 2 {
            w1059 = 57.0  # Level 3 PTO Okay
            w1061 = 62.0  # Level 3 Start
            w1073 = 60.0  # Level 3 PTO
            # "Level 3 buddy climb sequence"
            n355 = case shown="1" w1070 {
              selector: w1070 -> [w1084 w1100 w1116 w1134 w1146 w1168 w1182 w1195 w1215 w1224 w1237 w1249 w1267 w1280]
              tunnel: [w1086 w1102 w1111 w1133 w1145 w1167 w1181 w1194 w1214 w1223 w1236 w1248 w1266 w1280] -> w1064
              tunnel: [w1083 w1090 w1109 w1131 w1148 w1160 w1177 w1186 w1200 w1226 w1239 w1251 w1273 w1283] -> w1071
              tunnel: w1072 -> [_ w1090 w1109 _ w1148 w1160 w1177 _ w1200 w1226 w1239 w1251 w1273 w1283]
              tunnel: [w1082 w1099 w1122 w1132 w1144 w1170 w1184 w1197 w1217 w1227 w1240 w1252 w1274 w1284] -> w1065
              tunnel: [w1075 w1089 w1105 w1125 w1138 w1154 _ w1189 w1210 _ _ _ _ _] -> w1063
              tunnel: w1073 -> [_ _ _ _ _ _ w1174 w1189 w1210 _ _ _ _ _]
              tunnel: [w1080 w1098 w1110 w1129 w1143 w1163 w1180 w1193 w1213 w1228 w1241 w1253 w1275 w1285] -> w1066
              tunnel: [w1079 w1097 w1108 w1128 w1142 w1162 w1179 w1192 w1212 w1222 w1235 w1246 w1271 w1281] -> w1067
              tunnel: [FALSE FALSE FALSE FALSE FALSE FALSE FALSE FALSE FALSE FALSE TRUE TRUE TRUE FALSE] -> w1068
              tunnel: w1069 -> [_ _ _ _ _ _ _ _ _ _ _ _ _ _]
              tunnel: ["release mantis" "wait for mantis to deploy" "wait for elevator to reach climb height" "lock mantis" "confirm mantis lock" "wait for the driver to start climbing" "wait for elevator to pass PTO height" "engage the PTO" "ensure PTO is engaged" "wait for the robot to be on HAB" "stop climbing" "wait to disengage PTO" "retract the legs after confirm " "elevator powered down"] -> w1062
              tunnel: w1061 -> [_ _ w1105 w1125 w1138 w1154 _ _ _ _ _ _ _ _]
              tunnel: [-1.0 ("y") -1.0 ("y") -1.0 ("y") -1.0 ("y") -1.0 ("y") -1.0 ("y") -0.05 ("y") -0.05 ("y") -0.05 ("y") -1.0 ("y") -1.0 ("y") -1.0 ("y") -1.0 ("y") -1.0 ("y")] -> w1060
              tunnel: w1059 -> [_ _ _ _ _ _ _ _ w1206 _ _ _ _ _]
              tunnel: [_ _ _ _ _ _ _ _ _ _ _ _ _ w1277] -> w1058
              tunnel: w1057 -> [w1075 w1089 _ _ _ _ _ _ _ _ _ _ _ _]
              tunnel: [w1074 w1087 w1103 w1123 w1136 w1152 w1171 w1185 w1198 w1218 w1230 w1242 w1254 w1276] -> w1056
              frame 0, Default {
                w1074 = FALSE  # foot retracted
                w1079 = FALSE  # no PTO
                w1080 = FALSE  # not climbing
                w1082 = TRUE  # pins out
                # "release mantis pins and command to climb height"
                n356 = Increment(x=w1084) -> (x+1=w1085:i32)
                n357 = Select(t=w1085, s=TRUE, f=w1084) -> (s? t:f=w1086:i32)
                n358 = Tick Count (ms)() -> (millisecond timer value=w1083:u32)
              }
              frame 1 {
                w1087 = FALSE  # foot retracted
                w1097 = FALSE  # no PTO
                w1098 = FALSE  # not climbing
                w1099 = TRUE  # pins out
                # "wait for mantis to deploy"
                n359 = Tick Count (ms)() -> (millisecond timer value=w1093:u32)
                n360 = Subtract(x=w1093, y=w1090) -> (x-y=w1092:u32)
                n361 = Greater?(x=w1092, y=u32 250) -> (0:w1088:bool)
                n362 = Increment(x=w1100) -> (x+1=w1101:i32)
                n363 = Select(t=w1101, s=w1088, f=w1100) -> (s? t:f=w1102:i32)
              }
              frame 2 {
                w1103 = FALSE  # foot retracted
                w1108 = FALSE  # no PTO
                w1110 = FALSE  # not climbing
                w1122 = TRUE  # pins out
                # "wait for elevator to start moving\nand then stop moving"
                # "wait for elevator to reach climb position"
                n364 = global read "RobotStates.vi" "Elevator Moving"() -> (w1114:bool)
                n365 = call "RisingEdgeTrigger.vi"("Raw Signal"=w1114) -> ("Trigger"=w1121:bool)
                n366 = Not(x=w1114) -> (.not. x?=w1113:bool)
                n367 = feedback #19(FALSE) -> (w1119:bool)
                n368 = Select(t=TRUE, s=w1121, f=w1119) -> (s? t:f=w1115:bool)
                n369 = feedback-in #19(w1115) -> ()
                n370 = And(x=w1115, y=w1113) -> (x .and. y?=w1112:bool)
                n371 = Increment(x=w1116) -> (x+1=w1117:i32)
                n372 = Select(t=w1117, s=w1112, f=w1116) -> (s? t:f=w1111:i32)
              }
              frame 3 {
                w1123 = FALSE  # foot retracted
                w1128 = FALSE  # no PTO
                w1129 = FALSE  # not climbing
                w1132 = FALSE  # pins in
                # "lock mantis pins"
                n373 = Increment(x=w1134) -> (x+1=w1135:i32)
                n374 = Tick Count (ms)() -> (millisecond timer value=w1131:u32)
                n375 = Select(t=w1135, s=TRUE, f=w1134) -> (s? t:f=w1133:i32)
              }
              frame 4 {
                w1136 = FALSE  # foot retracted
                w1142 = FALSE  # no PTO
                w1143 = FALSE  # not climbing
                w1144 = FALSE  # pins in
                # "wait for mantis legs to lock"
                n376 = Tick Count (ms)() -> (millisecond timer value=w1151:u32)
                n377 = Subtract(x=w1151, y=w1148) -> (x-y=w1150:u32)
                n378 = Greater?(x=w1150, y=u32 500) -> (0:w1140:bool)
                n379 = Increment(x=w1146) -> (x+1=w1147:i32)
                n380 = Select(t=w1147, s=w1140, f=w1146) -> (s? t:f=w1145:i32)
              }
              frame 5 {
                w1152 = FALSE  # foot retracted
                w1162 = FALSE  # no PTO
                w1163 = FALSE  # not climbing
                w1170 = FALSE  # pins in
                # "wait for the driver to start climbing"
                n381 = global read "Inputs_DriverStation.vi" "J1-RightTrigger"() -> (w1159:dbl)
                n382 = Greater?(x=w1159, y=0.2) -> (0:w1157:bool)
                n383 = feedback #20(FALSE) -> (w1164:bool)
                n384 = Select(t=TRUE, s=w1157, f=w1164) -> (s? t:f=w1156:bool)
                n385 = feedback-in #20(w1156) -> ()
                n386 = Increment(x=w1168) -> (x+1=w1169:i32)
                n387 = Select(t=w1169, s=w1156, f=w1168) -> (s? t:f=w1167:i32)
              }
              frame 6 {
                w1171 = FALSE  # foot retracted
                w1179 = FALSE  # no PTO
                w1180 = TRUE  # climbing
                w1184 = FALSE  # pins in
                # "wait for elevator to pass PTO height"
                n388 = global read "SensorReadings.vi" "EncoderPos_Elevator"() -> (w1172:dbl)
                n389 = Less Or Equal?(x=w1172, y=w1174) -> (x <= y?=w1173:bool)
                n390 = Increment(x=w1182) -> (x+1=w1183:i32)
                n391 = Select(t=w1183, s=w1173, f=w1182) -> (s? t:f=w1181:i32)
              }
              frame 7 {
                w1185 = FALSE  # foot retracted
                w1192 = TRUE  # PTO
                w1193 = TRUE  # climbing
                w1197 = FALSE  # pins in
                # "engage the PTO"
                n392 = Increment(x=w1195) -> (x+1=w1196:i32)
                n393 = Tick Count (ms)() -> (millisecond timer value=w1186:u32)
                n394 = Select(t=w1196, s=TRUE, f=w1195) -> (s? t:f=w1194:i32)
              }
              frame 8 {
                w1198 = FALSE  # foot retracted
                w1212 = TRUE  # PTO
                w1213 = TRUE  # climbing
                w1217 = FALSE  # pins in
                # "timeout"
                # "ensure PTO is engaged"
                n395 = global read "SensorReadings.vi" "EncoderPos_Elevator"() -> (w1207:dbl)
                n396 = Tick Count (ms)() -> (millisecond timer value=w1203:u32)
                n397 = Less Or Equal?(x=w1207, y=w1206) -> (x <= y?=w1205:bool)
                n398 = Subtract(x=w1203, y=w1200) -> (x-y=w1202:u32)
                n399 = Greater?(x=w1202, y=u32 1000) -> (0:w1199:bool)
                n400 = Or(x=w1199, y=w1205) -> (x .or. y?=w1204:bool)
                n401 = Increment(x=w1215) -> (x+1=w1216:i32)
                n402 = Select(t=w1216, s=w1204, f=w1215) -> (s? t:f=w1214:i32)
              }
              frame 9 {
                w1218 = TRUE  # foot deployed
                w1222 = TRUE  # PTO
                w1228 = TRUE  # climbing
                w1227 = FALSE  # pins in
                # "wait for robot to be secure on HAB"
                n403 = global read "Inputs_DriverStation.vi" "J1-Menu"() -> (w1229:bool)
                n404 = Increment(x=w1224) -> (x+1=w1225:i32)
                n405 = Select(t=w1225, s=w1229, f=w1224) -> (s? t:f=w1223:i32)
              }
              frame 10 {
                w1230 = TRUE  # foot deployed
                w1235 = TRUE  # PTO
                w1241 = TRUE  # climbing
                w1240 = FALSE  # pins in
                # "******"
                # "stop \"climbing\""
                n406 = Increment(x=w1237) -> (x+1=w1238:i32)
                n407 = Select(t=w1238, s=TRUE, f=w1237) -> (s? t:f=w1236:i32)
              }
              frame 11 {
                w1242 = TRUE  # foot deployed
                w1246 = TRUE  # PTO
                w1253 = TRUE  # climbing
                w1252 = FALSE  # pins in
                # "******"
                # "wait to disengage PTO"
                n408 = Increment(x=w1249) -> (x+1=w1250:i32)
                n409 = Select(t=w1250, s=TRUE, f=w1249) -> (s? t:f=w1248:i32)
              }
              frame 12 {
                w1254 = TRUE  # foot deployed
                w1271 = FALSE  # no PTO
                w1275 = TRUE  # climbing
                w1274 = FALSE  # pins in
                # "*******"
                # "retract legs"
                n410 = global read "Inputs_DriverStation.vi" "J1-Menu"() -> (w1256:bool)
                n411 = Not(x=w1256) -> (.not. x?=w1257:bool)
                n412 = feedback #21(FALSE ("PTO")) -> (w1260:bool)
                n413 = Select(t=TRUE ("no PTO"), s=w1257, f=w1260) -> (s? t:f=w1255:bool)
                n414 = feedback-in #21(w1255) -> ()
                n415 = And(x=w1255, y=w1256) -> (x .and. y?=w1258:bool)
                n416 = feedback #22(FALSE ("PTO")) -> (w1264:bool)
                n417 = Select(t=TRUE ("no PTO"), s=w1258, f=w1264) -> (s? t:f=w1262:bool)
                n418 = feedback-in #22(w1262) -> ()
                n419 = Increment(x=w1267) -> (x+1=w1268:i32)
                n420 = Select(t=w1268, s=w1262, f=w1267) -> (s? t:f=w1266:i32)
              }
              frame 13 {
                w1276 = TRUE  # foot deployed
                w1277 = TRUE  # end of match
                w1281 = FALSE  # no PTO
                w1285 = TRUE  # climbing
                w1284 = FALSE  # pins in
                # "turn off the elevator"
              }
            }
          }
        }
      }
      n421 = feedback-in #8(w537) -> ()
      n422 = global write "RobotStates.vi" "Climb Sequence"(w532) -> ()
    }
  }
  "Target Elevator Position" <- w58
  "Target Vacuum Pump Power" <- w55
  n423 = feedback-in #5(w20) -> ()
  n424 = global write "RobotStates.vi" "Climb Sequence String"(w8) -> ()
  n425 = global write "SensorReadings.vi" "LimeLight In Range"(w5) -> ()
  n426 = global write "RobotStates.vi" "Climber Foot State"(w2) -> ()
  n427 = global write "SensorReadings.vi" "At HAB Height"(w9) -> ()
  n428 = global write "RobotStates.vi" "Max Climb Power"(w7) -> ()
  n429 = global write "RobotStates.vi" "End of Match"(w6) -> ()
  n430 = global write "RobotStates.vi" "PTO State"(w13) -> ()
  n431 = global write "RobotStates.vi" "Climb Started"(w14) -> ()
  n432 = global write "RobotStates.vi" "Climber Mantis State"(w1) -> ()
  n433 = global write "RobotStates.vi" "Upper Valve State"(w52) -> ()
  n434 = global write "RobotStates.vi" "Lower Valve State"(w51) -> ()
  n435 = global write "RobotStates.vi" "CARGO Intake Allowed"(w60) -> ()
  n436 = global write "RobotStates.vi" "CARGO Arm"(w59) -> ()
  n437 = global write "RobotStates.vi" "HATCH Arm"(w57) -> ()
  n438 = global write "RobotStates.vi" "HATCH Ejection Allowed"(w56) -> ()
  n439 = global read "Inputs_DriverStation.vi" "J1-View"() -> (w31:bool)
  n440 = Equal?(x=w29, y="Elevator_Stow") -> (x = y?=w45:bool)
  n441 = Equal?(x=w29, y="Cargo_Ground") -> (x = y?=w44:bool)
  n442 = Equal?(x=w29, y="Cargo_Feeder") -> (x = y?=w43:bool)
  n443 = Equal?(x=w29, y="Hatch_Ground") -> (x = y?=w42:bool)
  n444 = Equal?(x=w29, y="Hatch_Feeder") -> (x = y?=w41:bool)
  n445 = Equal?(x=w29, y="Climb") -> (x = y?=w40:bool)
  n446 = Compound Arithmetic op=OR(w45, w44, w43, w42, w41, w40, w31) -> (w37:bool)
  n447 = Not(x=w37) -> (.not. x?=w36:bool)
  n448 = while {
    shift-right: [w1290] -> w30
    shift-left: _ -> [w1291]
    tunnel: w36 -> [w1289]
    shift-right: [w1288] -> _
    shift-left: _ -> [w1287]
    tunnel: w29 -> [w1286]
    tunnel: [w1286] -> w28
    stop <- TRUE stop-if-true
    n449 = case shown="True" w1289 {
      tunnel: w1291 -> [_ w1298]
      tunnel: [0 w1297] -> w1290
      tunnel: [w1293 w1296] -> w1288
      tunnel: w1287 -> [w1293 w1295]
      frame False {
        # "stow, ground pickup, or feeder station"
      }
      frame True {
        # "rocket are cargo ship"
        n450 = case shown="1" w1298 {
          selector: w1298 -> [w1301 w1309 w1323 w1334 w1338 _]
          tunnel: [w1300 w1311 w1318 w1335 w1337 0 ("t")] -> w1297
          tunnel: [w1299 w1308 w1316 w1328 w1336 w1344] -> w1296
          tunnel: w1295 -> [w1299 _ w1316 _ w1336 w1344]
          frame 0, Default {
            # "wait for driver to start release"
            n451 = global read "Inputs_DriverStation.vi" "J1-LeftTrigger"() -> (w1304:dbl)
            n452 = Greater?(x=w1304, y=0.75) -> (0:w1302:bool)
            n453 = Increment(x=w1301) -> (x+1=w1305:i32)
            n454 = Select(t=w1305, s=w1302, f=w1301) -> (s? t:f=w1300:i32)
          }
          frame 1 {
            # "check for game piece release"
            n455 = global read "SensorReadings.vi" "Hatch Captured"() -> (w1314:bool)
            n456 = global read "SensorReadings.vi" "Cargo Captured"() -> (w1313:bool)
            n457 = Not(x=w1313) -> (.not. x?=w1307:bool)
            n458 = Not(x=w1314) -> (.not. x?=w1306:bool)
            n459 = Or(x=w1306, y=w1307) -> (x .or. y?=w1312:bool)
            n460 = Increment(x=w1309) -> (x+1=w1310:i32)
            n461 = Tick Count (ms)() -> (millisecond timer value=w1308:u32)
            n462 = Select(t=w1310, s=w1312, f=w1309) -> (s? t:f=w1311:i32)
          }
          frame 2 {
            # "***200"
            # "check to see if game piece actually gone"
            n463 = global read "SensorReadings.vi" "Hatch Captured"() -> (w1320:bool)
            n464 = global read "SensorReadings.vi" "Cargo Captured"() -> (w1321:bool)
            n465 = Tick Count (ms)() -> (millisecond timer value=w1327:u32)
            n466 = Subtract(x=w1327, y=w1316) -> (x-y=w1326:u32)
            n467 = Greater?(x=w1326, y=u32 0) -> (0:w1324:bool)
            n468 = Or(x=w1320, y=w1321) -> ()  [unwired: 1 out]
            n469 = Increment(x=w1323) -> (x+1=w1322:i32)
            n470 = Select(t=w1322, s=w1324, f=w1323) -> (s? t:f=w1319:i32)
            n471 = Select(t=0, s=FALSE, f=w1319) -> (s? t:f=w1318:i32)
          }
          frame 3 {
            # "wait for driver to release trigger"
            n472 = global read "Inputs_DriverStation.vi" "J1-LeftTrigger"() -> (w1332:dbl)
            n473 = Greater?(x=w1332, y=0.1) -> (0:w1330:bool)
            n474 = Not(x=w1330) -> (.not. x?=w1329:bool)
            n475 = Increment(x=w1334) -> (x+1=w1333:i32)
            n476 = Select(t=w1333, s=w1329, f=w1334) -> (s? t:f=w1335:i32)
            n477 = Tick Count (ms)() -> (millisecond timer value=w1328:u32)
          }
          frame 4 {
            # "safety wait"
            n478 = Tick Count (ms)() -> (millisecond timer value=w1343:u32)
            n479 = Subtract(x=w1343, y=w1336) -> (x-y=w1342:u32)
            n480 = Greater?(x=w1342, y=u32 50) -> (0:w1340:bool)
            n481 = Increment(x=w1338) -> (x+1=w1339:i32)
            n482 = Select(t=w1339, s=w1340, f=w1338) -> (s? t:f=w1337:i32)
          }
          frame 5 {
            # "trigger auto stow"
            n483 = global write "RobotStates.vi" "Auto Stow"(TRUE) -> ()
          }
        }
      }
    }
  }
  "Elevator State Out" <- w28
  n484 = global write "RobotStates.vi" "Auto Stow Sequence"(w30) -> ()
